vi "Start All.vi"(8 "error in (no error)":errorcluster, 11 "Thread Manager in":refnum<class "Thread Manager.lvclass">) -> (0 "error out":errorcluster, 3 "Thread Manager out":refnum<class "Thread Manager.lvclass">)   [LabVIEW 2017, in "DSF Core.lvlib" / "Thread Manager.lvclass"]
uses:
  Thread Manager.lvclass
  Thread/DSF Thread Options.ctl
  Thread Manager.lvclass/Thread Manager.ctl
  Thread/Thread.lvclass
  DSF Core.lvlib
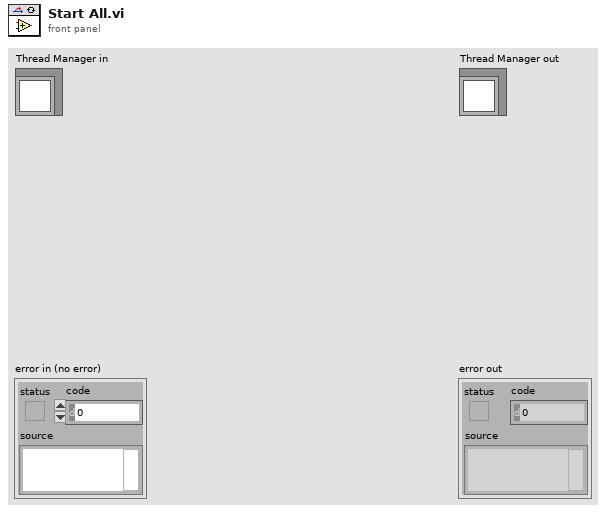
[diagram p1: front panel]
types:
  T1 = typedef "DSF Core.lvlib/DSF Thread Options.ctl" = cluster{"Show FP On Call":bool, "Close FP After Call":bool, "Allow Debugging":bool}
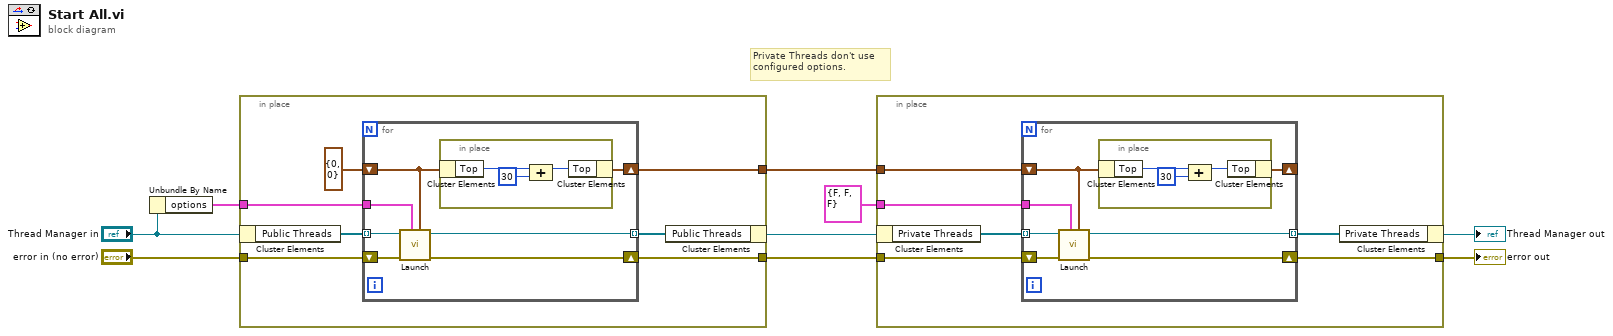
[diagram p0: block diagram]
diagram:
  # "Private Threads don't use configured options."
  n1 = Unbundle By Name("Thread Manager in") -> ("options"=w9:T1)
  n2 = in-place {
    in-place-border: [w14] -> w4
    in-place-border: "error in (no error)" -> [w13]
    in-place-border: w9 -> [w11]
    in-place-border: [w10] -> w1
    n3 = in-place-cluster #1("Thread Manager in") -> ("Public Threads"=w16:refnum<class "Thread.lvclass">[])
    n4 = for {
      tunnel: w16 -> [w23] mode=indexing
      tunnel: [w22] -> w15 mode=indexing
      shift-right: [w20] -> w14
      shift-left: w13 -> [w21]
      shift-right: [w18] -> w10
      shift-left: cluster{"Left":i16, "Top":i16} {"Left"=0, "Top"=0} ("window position") -> [w19]
      tunnel: w11 -> [w17]
      n5 = call "Launch.vi"("window position"=w19, "options"=w17, "error in (no error)"=w21, "Thread in"=w23) -> ("error out"=w20:errorcluster, "Thread out"=w22:refnum<class "Thread.lvclass">)  [unwired: 6 in]
      n6 = in-place {
        n7 = in-place-cluster #2(w19) -> ("Top"=w26:i16)
        n8 = Compound Arithmetic op=ADD(w26, i16 30 ("y")) -> (w24:i16)
        n9 = in-place-cluster #2("Top"=w24) -> (w18:cluster{"Left":i16, "Top":i16})
      }
    }
    n10 = in-place-cluster #1("Public Threads"=w15) -> (w5:refnum<class "Thread Manager.lvclass">)
  }
  n11 = in-place {
    in-place-border: [w30] -> w2
    in-place-border: w4 -> [w29]
    in-place-border: T1 {"Show FP On Call"=FALSE, "Close FP After Call"=FALSE, "Allow Debugging"=FALSE} ("options") -> [w28]
    in-place-border: w1 -> [w27]
    n12 = in-place-cluster #3(w5) -> ("Private Threads"=w32:refnum<class "Thread.lvclass">[])
    n13 = for {
      tunnel: w32 -> [w39] mode=indexing
      tunnel: [w38] -> w31 mode=indexing
      shift-right: [w36] -> w30
      shift-left: w29 -> [w37]
      shift-right: [w34] -> _
      shift-left: w27 -> [w35]
      tunnel: w28 -> [w33]
      n14 = call "Launch.vi"("window position"=w35, "options"=w33, "error in (no error)"=w37, "Thread in"=w39) -> ("error out"=w36:errorcluster, "Thread out"=w38:refnum<class "Thread.lvclass">)  [unwired: 6 in]
      n15 = in-place {
        n16 = in-place-cluster #4(w35) -> ("Top"=w42:i16)
        n17 = Compound Arithmetic op=ADD(w42, i16 30 ("y")) -> (w40:i16)
        n18 = in-place-cluster #4("Top"=w40) -> (w34:cluster{"Left":i16, "Top":i16})
      }
    }
    n19 = in-place-cluster #3("Private Threads"=w31) -> (→"Thread Manager out":refnum<class "Thread Manager.lvclass">)
  }
  "error out" <- w2
